vi "response_interpreter.vi"(1 "Response type":u16(ring) items=["String", "Integer", "Long", "Float", "Byte", "Bits"], 2 "Response hex":string) -> (0 "Response (readable)":string)   [LabVIEW 2012]
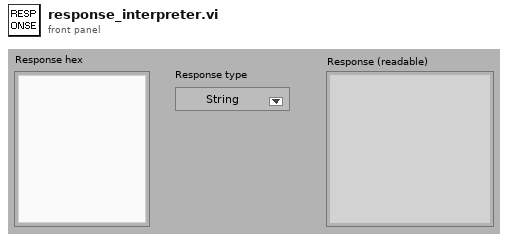
[diagram p1: front panel]
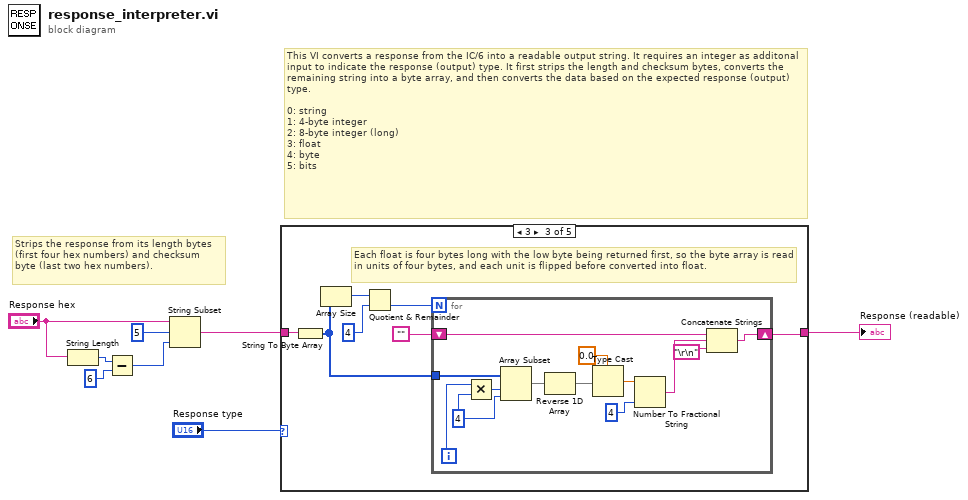
[diagram p0: block diagram]
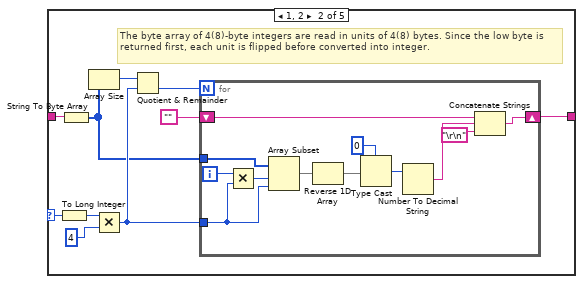
[diagram p3: hidden frame]
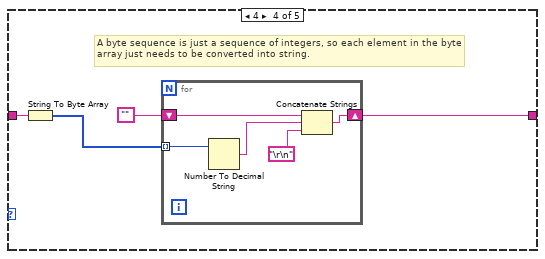
[diagram p4: hidden frame]
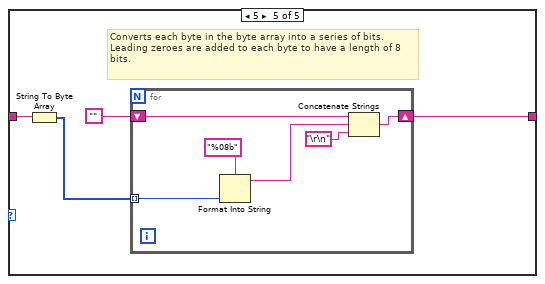
[diagram p5: hidden frame]
diagram:
  # "Strips the response from its length bytes (first four hex numbers) and checksum byte (last two hex numbers)."
  # "This VI converts a response from the IC/6 into a readable output string. It requires an integer as additonal input to indicate the response (output) type. It first strips the length and checksum bytes, converts the remaining string into a byte array, and then converts the data based on the expected response (output) type.\n\n0: string\n1: 4-byte integer\n2: 8-byte integer (long)\n3: float\n4: byte\n5: bits"
  n1 = String Length(string="Response hex") -> (length=w6:i32)
  n2 = Subtract(x=w6, y=6) -> (x-y=w4:i32)
  n3 = String Subset(string="Response hex", offset (0)=5, length (rest)=w4) -> (substring=w1:string)
  n4 = case shown="3" "Response type" {
    selector: "Response type" -> [_ w17 _ _ _]
    tunnel: [w9 w18 w36 w54 w63] -> w3
    tunnel: w1 -> [w9 w14 w35 w53 w62]
    frame 0, Default {
      # "Output is string, so no special treatment is required."
    }
    frame 1, 2 {
      # "The byte array of 4(8)-byte integers are read in units of 4(8) bytes. Since the low byte is returned first, each unit is flipped before converted into integer."
      n5 = To Long Integer(number=w17) -> (32bit integer=w12:i32)
      n6 = String To Byte Array(string=w14) -> (unsigned byte array=w13:u8[])
      n7 = Array Size(array=w13) -> (size(s)=w10:i32)
      n8 = Multiply(x=w12, y=4) -> (x*y=w16:i32)
      n9 = Quotient & Remainder(x=w10, y=w16) -> (floor(x/y)=w11:i32)  [unwired: 1 out]
      n10 = for {
        N: w11 -> [_]
        tunnel: w13 -> [w23]
        shift-right: [w27] -> w18
        shift-left: "" -> [w28]
        tunnel: w16 -> [w20]
        i -> [w22]
        n11 = Multiply(x=w22, y=w20) -> (x*y=w21:i32)
        n12 = Array Subset(array=w23, index=w21, length=w20) -> (w24:u8[])
        n13 = Reverse 1D Array(array=w24) -> (reversed array=w29:u8[])
        n14 = Type Cast(type=0, x=w29) -> (*(type *) &x=w30:i32)
        n15 = Number To Decimal String(number=w30) -> (decimal integer string=w25:string)  [unwired: 1 in]
        n16 = Concatenate Strings(w28, w25, "\r\n") -> (w27:string)
      }
    }
    frame 3 {
      # "Each float is four bytes long with the low byte being returned first, so the byte array is read in units of four bytes, and each unit is flipped before converted into float."
      n17 = String To Byte Array(string=w35) -> (unsigned byte array=w34:u8[])
      n18 = Array Size(array=w34) -> (size(s)=w32:i32)
      n19 = Quotient & Remainder(x=w32, y=4) -> (floor(x/y)=w33:i32)  [unwired: 1 out]
      n20 = for {
        N: w33 -> [_]
        tunnel: w34 -> [w43]
        shift-right: [w47] -> w36
        shift-left: "" -> [w48]
        i -> [w42]
        w40 = 4
        n21 = Multiply(x=w42, y=w40) -> (x*y=w41:i32)
        n22 = Array Subset(array=w43, index=w41, length=w40) -> (w44:u8[])
        n23 = Reverse 1D Array(array=w44) -> (reversed array=w49:u8[])
        n24 = Type Cast(type=sgl 0.0, x=w49) -> (*(type *) &x=w50:sgl)
        n25 = Number To Fractional String(number=w50, precision (6)=4) -> (F-format string=w45:string)  [unwired: 2 in]
        n26 = Concatenate Strings(w48, w45, "\r\n") -> (w47:string)
      }
    }
    frame 4 {
      # "A byte sequence is just a sequence of integers, so each element in the byte array just needs to be converted into string."
      n27 = String To Byte Array(string=w53) -> (unsigned byte array=w52:u8[])
      n28 = for {
        shift-right: [w58] -> w54
        shift-left: "" -> [w59]
        tunnel: w52 -> [w57] mode=indexing
        n29 = Number To Decimal String(number=w57) -> (decimal integer string=w56:string)  [unwired: 1 in]
        n30 = Concatenate Strings(w59, w56, "\r\n") -> (w58:string)
      }
    }
    frame 5 {
      # "Converts each byte in the byte array into a series of bits. Leading zeroes are added to each byte to have a length of 8 bits."
      n31 = String To Byte Array(string=w62) -> (unsigned byte array=w61:u8[])
      n32 = for {
        tunnel: w61 -> [w70] mode=indexing
        shift-right: [w69] -> w63
        shift-left: "" -> [w68]
        n33 = Format Into String(format string="%08b", w70) -> (resulting string=w67:string)  [unwired: 2 in, 1 out]
        n34 = Concatenate Strings(w68, w67, "\r\n") -> (w69:string)
      }
    }
  }
  "Response (readable)" <- w3
